vi "SerialNo.vi"() -> (2 "Continue?":bool)   [LabVIEW 2018]
uses:
  globals/QC_RunInformation.vi
panel:
  in  "DB Serial No.:":string
  in  "Batch No.:":string
  in  "Device Category:":string(combo)="Short Strip"
  in  "Manufacturer:":string(combo)="Hamamatsu"
  in  "Wafer Serial No.:":string
  in  "Sensor Serial No.:":string
  in  "Cancel":bool
  in  "OK":bool
  in  "Barcode reader":bool
  # "ATLAS Serial No."
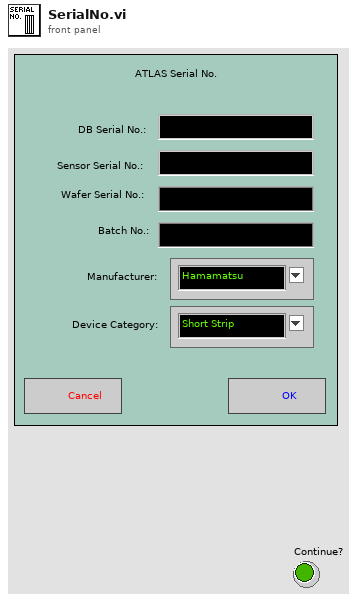
[diagram p1: front panel]
types:
  T1 = cluster{"Sensor Serial No.:":string, "Wafer Serial No.:":string, "Batch:":string, "Manufacturer:":string, "Device Category:":string, "Database Serial No.:":string, "Initiated:":string, "Test":string, "Instruments used:":string, "Probeplan used:":string, "End of Run comment:":string, "User:":string}
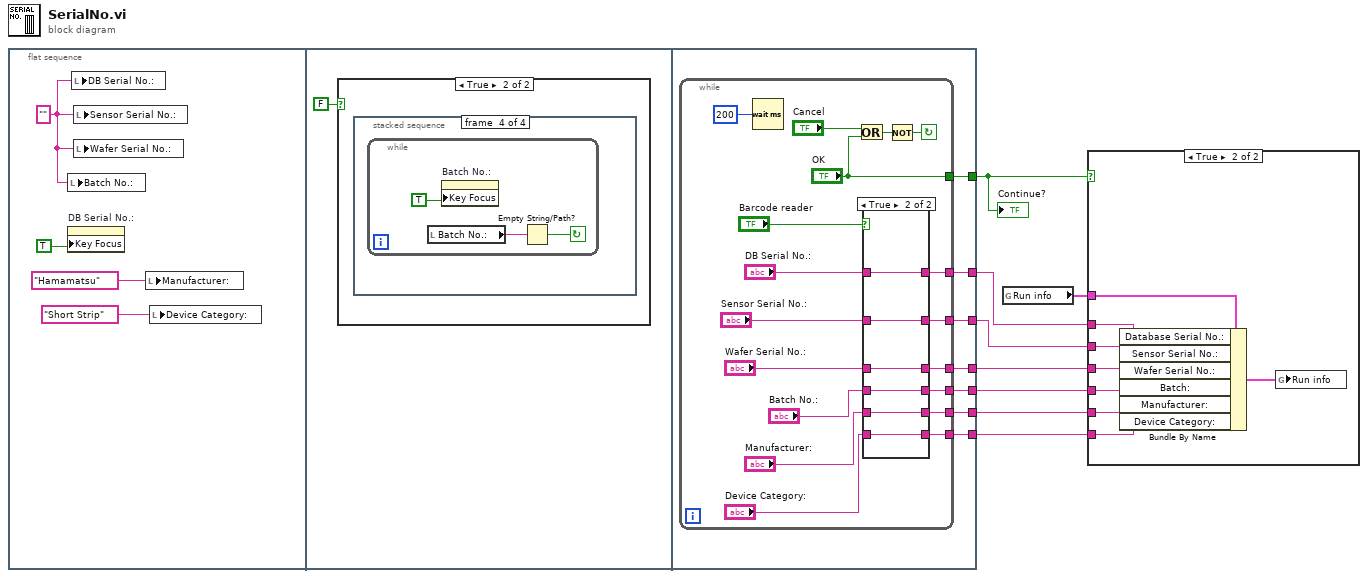
[diagram p0: block diagram]
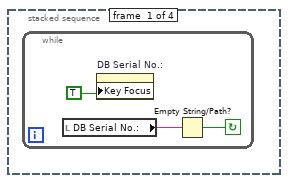
[diagram p4: hidden frame]
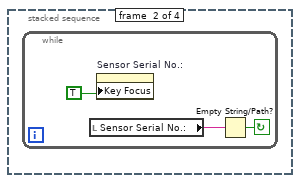
[diagram p5: hidden frame]
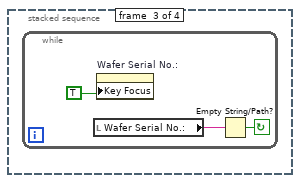
[diagram p6: hidden frame]
diagram:
  n1 = flat-sequence {
    tunnel: [w32] -> w8
    tunnel: [w31] -> w2
    tunnel: [w30] -> w6
    tunnel: [w29] -> w7
    tunnel: [w28] -> w1
    tunnel: [w27] -> w4
    tunnel: [w26] -> w3
    frame #0 {
      w11 = ""
      n2 = local write "Batch No.:"(w11) -> ()
      n3 = property on="DB Serial No.:" class="Str"("Key Focus"=TRUE) -> ()  [unwired: 2 in, 2 out]
      n4 = local write "DB Serial No.:"(w11) -> ()
      n5 = local write "Sensor Serial No.:"(w11) -> ()
      n6 = local write "Wafer Serial No.:"(w11) -> ()
      n7 = local write "Manufacturer:"("Hamamatsu" ("Manufacturer:")) -> ()
      n8 = local write "Device Category:"("Short Strip" ("Device Category:")) -> ()
    }
    frame #1 {
      n9 = case shown="True" FALSE {
        frame False {
        }
        frame True {
          n10 = stacked-sequence {
            frame #0 {
              n11 = while {
                stop <- w14 continue-if-true
                n12 = local read "DB Serial No.:"() -> (w15:string)
                n13 = property on="DB Serial No.:" class="Str"("Key Focus"=TRUE) -> ()  [unwired: 2 in, 2 out]
                n14 = Empty String/Path?(string/path=w15) -> (empty?=w14:bool)
              }
            }
            frame #1 {
              n15 = while {
                stop <- w18 continue-if-true
                n16 = local read "Sensor Serial No.:"() -> (w17:string)
                n17 = property on="Sensor Serial No.:" class="Str"("Key Focus"=TRUE) -> ()  [unwired: 2 in, 2 out]
                n18 = Empty String/Path?(string/path=w17) -> (empty?=w18:bool)
              }
            }
            frame #2 {
              n19 = while {
                stop <- w21 continue-if-true
                n20 = local read "Wafer Serial No.:"() -> (w20:string)
                n21 = property on="Wafer Serial No.:" class="Str"("Key Focus"=TRUE) -> ()  [unwired: 2 in, 2 out]
                n22 = Empty String/Path?(string/path=w20) -> (empty?=w21:bool)
              }
            }
            frame #3 {
              n23 = while {
                stop <- w24 continue-if-true
                n24 = local read "Batch No.:"() -> (w23:string)
                n25 = property on="Batch No.:" class="Str"("Key Focus"=TRUE) -> ()  [unwired: 2 in, 2 out]
                n26 = Empty String/Path?(string/path=w23) -> (empty?=w24:bool)
              }
            }
          }
        }
      }
    }
    frame #2 {
      n27 = while {
        tunnel: ["OK"] -> w31
        tunnel: [w43] -> w28
        tunnel: [w44] -> w32
        tunnel: [w42] -> w27
        tunnel: [w41] -> w26
        tunnel: [w40] -> w30
        tunnel: [w39] -> w29
        stop <- w48 continue-if-true
        n28 = Wait (ms)(milliseconds to wait=200) -> ()  [unwired: 1 out]
        n29 = Or(x="Cancel", y="OK") -> (x .or. y?=w49:bool)
        n30 = case shown="True" "Barcode reader" {
          tunnel: "DB Serial No.:" -> [w56 w62]
          tunnel: "Sensor Serial No.:" -> [w55 w61]
          tunnel: "Wafer Serial No.:" -> [w54 w60]
          tunnel: [w56 w62] -> w44
          tunnel: [w55 w61] -> w43
          tunnel: [w54 w60] -> w42
          tunnel: "Batch No.:" -> [w53 w59]
          tunnel: [w53 w59] -> w41
          tunnel: "Manufacturer:" -> [w52 w58]
          tunnel: [w52 w58] -> w40
          tunnel: "Device Category:" -> [w51 w57]
          tunnel: [w51 w57] -> w39
          frame False {
          }
          frame True {
          }
        }
        n31 = Not(x=w49) -> (.not. x?=w48:bool)
      }
    }
  }
  n32 = global read "QC_RunInformation.vi" "Run info"() -> (w5:T1)
  n33 = case shown="True" w2 {
    tunnel: w8 -> [_ w70]
    tunnel: w7 -> [_ w69]
    tunnel: w6 -> [_ w68]
    tunnel: w5 -> [_ w67]
    tunnel: w4 -> [_ w66]
    tunnel: w3 -> [_ w65]
    tunnel: w1 -> [_ w63]
    frame False {
    }
    frame True {
      n34 = Bundle By Name(cluster=w67, "Database Serial No.:"=w70, "Sensor Serial No.:"=w63, "Wafer Serial No.:"=w66, "Batch:"=w65, "Manufacturer:"=w68, "Device Category:"=w69) -> (w64:T1)
      n35 = global write "QC_RunInformation.vi" "Run info"(w64) -> ()
    }
  }
  "Continue?" <- w2
